vi "OAT Single Stage Decimation with IC.vi"(6 "initial state":dbl[](array[numeric]) format="%.2f", 8 "error in (no error)":errorcluster, 9 "filter":T1={"coefficients"=[], "factor"=1} {"coefficients" format="%.2f"}, 11 "X":dbl[](array[numeric]) format="%.2f") -> (0 "error out":errorcluster, 3 "Y":dbl[](array[numeric]) format="%.2f", 4 "final state":dbl[](array[numeric]) format="%.2f")   [LabVIEW 2017, in "SoundVib_Resampling.lvlib"]
doc: "Decimate the input sequence <B>X</B> with the single stage decimation filter specified by <B>filter</B>."
uses:
  <vilib>/addons/Sound and Vibration/Order Analysis/Resample Order Tracking/SoundVib_Resampling.lvlib
  <vilib>/addons/_NISVFA/_Shared subVIs/Controls/OAT Decimation Filter.ctl
  <resource>/sndvib.dll
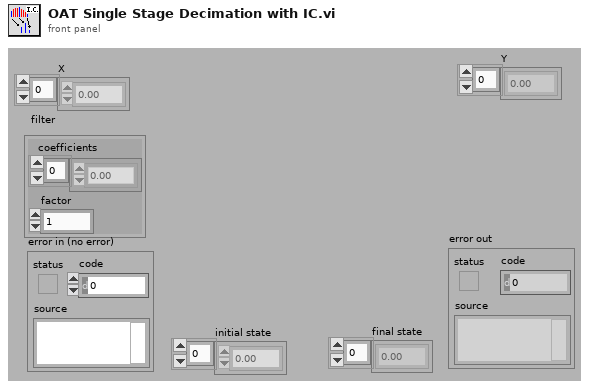
[diagram p1: front panel]
types:
  T1 = typedef "OAT Decimation Filter.ctl" = cluster{"coefficients":dbl[], "factor":i32}
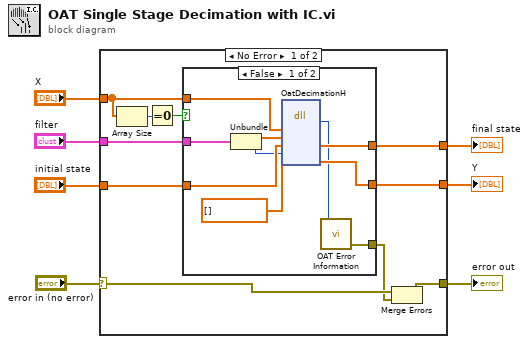
[diagram p0: block diagram]
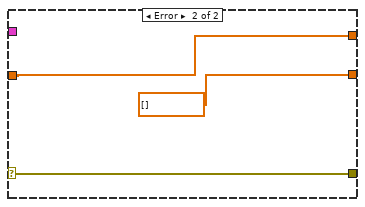
[diagram p3: hidden frame]
diagram:
  n1 = case shown="No Error" "error in (no error)" {
    selector: "error in (no error)" -> [w10 w32]
    tunnel: "initial state" -> [w17 w31]
    tunnel: [w16 w31] -> w6
    tunnel: "X" -> [w13 _]
    tunnel: [w15 dbl[] [] ("yH")] -> w4
    tunnel: "filter" -> [w14 _]
    tunnel: [w8 w32] -> w1
    frame No Error {
      n2 = Array Size(array=w13) -> (size(s)=w12:i32)
      n3 = Equal To 0?(x=w12) -> (x = 0?=w11:bool)
      n4 = case shown="False" w11 {
        tunnel: w17 -> [w27 w28]
        tunnel: [w26 w28] -> w16
        tunnel: [w25 w29] -> w15
        tunnel: w14 -> [w24 _]
        tunnel: [w19 _] -> w9
        tunnel: w13 -> [w18 w29]
        frame False {
          n5 = Unbundle(w24) -> ("coefficients"=w23:dbl[], "factor"=w22:i32)
          n6 = dll-call lib="C:/Program Files (x86)/National Instruments/LabVIEW 2017/resource/sndvib.*" fn="OatDecimationH"("xH"=w18, "filterH"=w23, "initH"=w27, "dec_factor"=w22, "yH"=dbl[] []) -> ("return type"=w20:i32, "initH"=w26:dbl[], "yH"=w25:dbl[])  [unwired: 6 in, 2 out]
          n7 = call <vilib>:"OAT Error Information.vi"("error code"=w20) -> ("error out"=w19:errorcluster)  [unwired: 6 in]
        }
        frame True {
        }
      }
      n8 = Merge Errors(w10, w9) -> (w8:errorcluster)
    }
    frame Error {
    }
  }
  "final state" <- w6
  "Y" <- w4
  "error out" <- w1
